vi "Untitled 2.vi"() -> ()   [LabVIEW 2017]
uses:
  <vilib>/NI/JSON Support for LabVIEW/JSON Value/New JSON Value/New JSON (String[]).vi
  <vilib>/NI/JSON Support for LabVIEW/JSON Value/JSON Value.lvclass
panel:
  out "x-y":u32
  out "Array":string[](array[string])
  out "16bit integer":u16[](array[numeric])
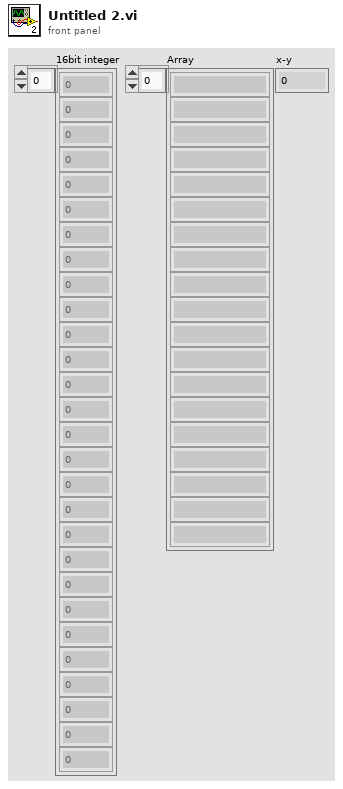
[diagram p1: front panel]
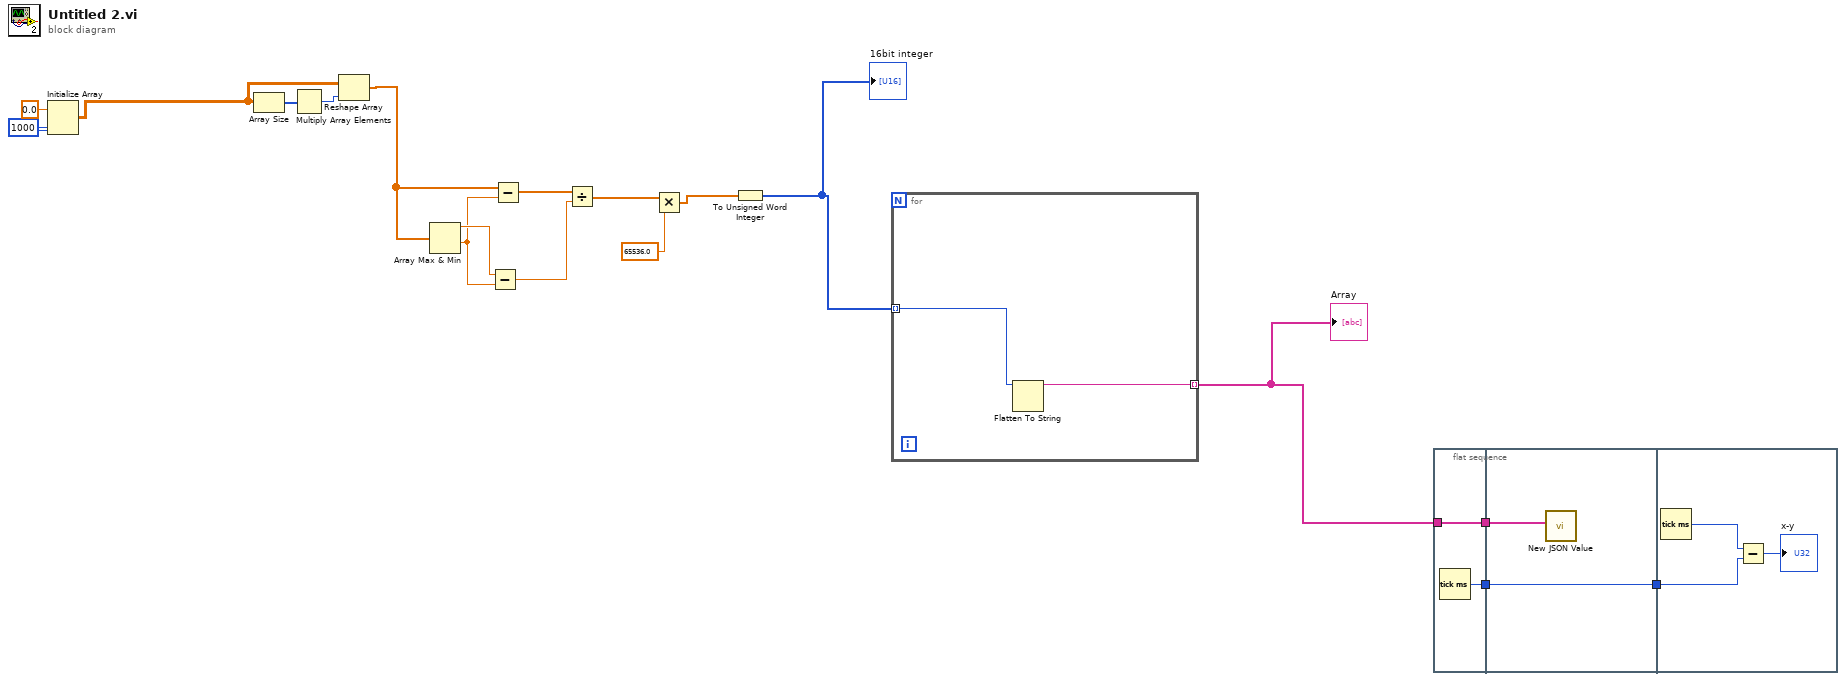
[diagram p0: block diagram]
diagram:
  w6 = 1000 ("dimension size")
  n1 = Initialize Array(0.0 ("element"), w6, w6) -> (w5:dbl[][])
  n2 = Array Size(array=w5) -> (size(s)=w17:i32[])
  n3 = Multiply Array Elements(1:w17) -> (0:w18:i32)
  n4 = Reshape Array(w5, w18) -> (w16:dbl[])
  n5 = Array Max & Min(array=w16) -> (max value=w14:dbl, min value=w13:dbl)  [unwired: 2 out]
  n6 = Subtract(x=w14, y=w13) -> (x-y=w12:dbl)
  n7 = Subtract(x=w16, y=w13) -> (x-y=w15:dbl[])
  n8 = Divide(x=w15, y=w12) -> (x/y=w11:dbl[])
  n9 = Multiply(x=w11, y=65536.0) -> (x*y=w9:dbl[])
  n10 = To Unsigned Word Integer(number=w9) -> (unsigned 16bit integer=w8:u16[])
  "16bit integer" <- w8
  n11 = for {
    tunnel: w8 -> [w19] mode=indexing
    tunnel: [w20] -> w4 mode=indexing
    n12 = Flatten To String(anything=w19) -> (data string=w20:string)  [unwired: 3 in, 2 out]
  }
  "Array" <- w4
  n13 = flat-sequence {
    tunnel: w4 -> [w22]
    tunnel: [w22] -> w3
    tunnel: [w21] -> w2
    tunnel: w3 -> [w24]
    tunnel: w2 -> [w23]
    tunnel: [w23] -> w1
    tunnel: w1 -> [w26]
    frame #0 {
      n14 = Tick Count (ms)() -> (millisecond timer value=w21:u32)
    }
    frame #1 {
      n15 = call-poly <vilib>:"New JSON Value.vi"("String Array"=w24) -> ()  [unwired: 9 in, 2 out]
    }
    frame #2 {
      n16 = Tick Count (ms)() -> (millisecond timer value=w27:u32)
      n17 = Subtract(x=w27, y=w26) -> (x-y=→"x-y":u32)
    }
  }
